vi "Autonomous Independent.vi"   [LabVIEW 2014]
doc: "This VI is called when autonomous begins, and will automatically be terminated when autonomous ends. You can carry out timed or sensor driven robot movement independently without needing to return to the caller."
uses:
  Robot Global Data.vi
panel:
  # "Be sure to right-click and choose Data Operations>>Make Current Value default if you want to save the array values with the VI"
types:
  T1 = enum16{"Nothing", "Load", "Lock", "Pass", "Grab", "Loader Down", "Shoot", "Auto Start", "Tele Start"}
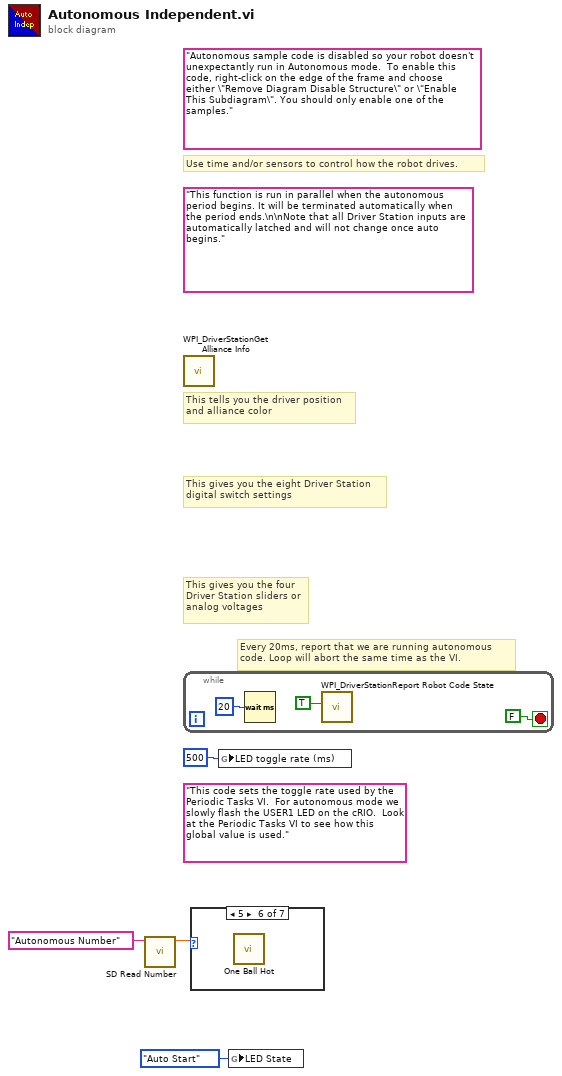
[diagram p0: block diagram]
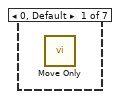
[diagram p2: hidden frame]
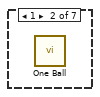
[diagram p3: hidden frame]
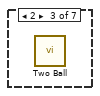
[diagram p4: hidden frame]
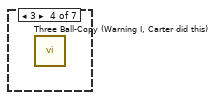
[diagram p5: hidden frame]
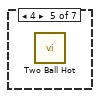
[diagram p6: hidden frame]
diagram:
  (unwired) "This code sets the toggle rate used by the Periodic Tasks VI.  For autonomous mode we slowly flash the USER1 LED on the cRIO.  Look at the Periodic Tasks VI to see how this global value is used."
  (unwired) "Autonomous sample code is disabled so your robot doesn't unexpectantly run in Autonomous mode.  To enable this code, right-click on the edge of the frame and choose either \"Remove Diagram Disable Structure\" or \"Enable This Subdiagram\". You should only enable one of the samples."
  (unwired) "This function is run in parallel when the autonomous period begins. It will be terminated automatically when the period ends.\n\nNote that all Driver Station inputs are automatically latched and will not change once auto begins."
  # "Every 20ms, report that we are running autonomous\ncode. Loop will abort the same time as the VI."
  # "Use time and/or sensors to control how the robot drives."
  # "This tells you the driver position\nand alliance color"
  # "This gives you the eight Driver Station\ndigital switch settings"
  # "This gives you the four\nDriver Station sliders or\nanalog voltages"
  n1 = call <vilib>:"SD Read Number.vi"("Name"="Autonomous Number") -> ("Numeric"=w2:dbl)  [unwired: 8 in, 2 out]
  n2 = call <vilib>:"WPI_DriverStationGet Alliance Info.vi"() -> ()  [unwired: 12 out]
  n3 = while {
    stop <- FALSE stop-if-true
    n4 = Wait (ms)(milliseconds to wait=u32 20) -> ()  [unwired: 1 out]
    n5 = call <vilib>:"WPI_DriverStationReport Robot Code State.vi"("Autonomous"=TRUE) -> ()  [unwired: 10 in, 1 out]
  }
  n6 = case shown="5" w2 {
    frame 0, Default {
      n7 = call "Move Only.vi"() -> ()  [unwired: 12 in]
    }
    frame 1 {
      n8 = call "One Ball.vi"() -> ()  [unwired: 12 in]
    }
    frame 2 {
      n9 = call "Two Ball.vi"() -> ()  [unwired: 12 in]
    }
    frame 3 {
      n10 = call "Three Ball-Copy (Warning I, Carter did this).vi"() -> ()  [unwired: 12 in]
    }
    frame 4 {
      n11 = call "Two Ball Hot.vi"() -> ()  [unwired: 12 in]
    }
    frame 5 {
      n12 = call "One Ball Hot.vi"() -> ()  [unwired: 12 in]
    }
    frame 6 {
    }
  }
  n13 = global write "Robot Global Data.vi" "LED toggle rate (ms)"(u32 500 ("LED ms toggle rate")) -> ()
  n14 = global write "Robot Global Data.vi" "LED State"(T1."Auto Start" ("LED State")) -> ()
